vi "Bitmap File Writer.vi"   [LabVIEW 2012]
panel:
  # "观察程序框图，运行本VI。\n\n本VI没有用户界面项。"
types:
  T1 = enum16{"open", "replace", "create", "open or create", "replace or create", "replace or create with confirmation"}
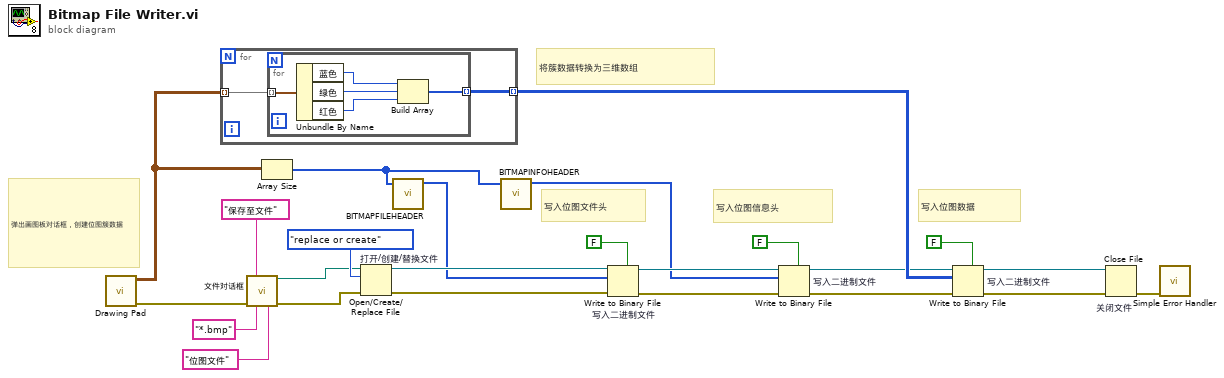
[diagram p0: block diagram]
diagram:
  # "弹出画图板对话框，创建位图簇数据"
  # "将簇数据转换为三维数组"
  # "写入位图数据"
  # "写入位图信息头"
  # "写入位图文件头"
  n1 = call "Drawing Pad.vi"() -> ("错误输出"=w4:errorcluster, "图像数据"=w14:cluster{"红色":u8, "绿色":u8, "蓝色":u8}[][])  [unwired: 10 in]
  n2 = for {
    tunnel: w14 -> [w26] mode=indexing
    tunnel: [w25] -> w12 mode=indexing
    n3 = for {
      tunnel: w26 -> [w31] mode=indexing
      tunnel: [w27] -> w25 mode=indexing
      n4 = Unbundle By Name ("按名称解除捆绑")(w31) -> ("蓝色"=w29:u8, "绿色"=w30:u8, "红色"=w28:u8)
      n5 = Build Array ("创建数组")(w29, w30, w28) -> (w27:u8[])
    }
  }
  n6 = call "文件对话框"("prompt"="保存至文件" ("提示"), "error in"=w4, "pattern (all files)"="*.bmp" ("类型（所有文件）"), "pattern label"="位图文件" ("类型标签")) -> ("selected path"=w6:path, "error out"=w5:errorcluster)  [unwired: 8 in, 2 out]
  n7 = Array Size ("数组大小")(array=w14) -> (size(s)=w17:i32[])
  n8 = Open/Create/Replace File "打开/创建/替换文件"(file path (use dialog)=w6, error in=w5, operation (0:open)=T1."replace or create" ("操作(0:open)")) -> (refnum out=w21:refnum<file>, error out=w20:errorcluster)  [unwired: 3 in, 1 out]
  n9 = call "BITMAPFILEHEADER.vi"("图像维数"=w17) -> ("位图文件头"=w16:u8[])  [unwired: 10 in]
  n10 = call "BITMAPINFOHEADER.vi"("图像维数"=w17) -> ("位图文件头"=w15:u8[])  [unwired: 10 in]
  n11 = Write to Binary File "写入二进制文件"(file (use dialog)=w21, data=w16, error in=w20, 5:FALSE ("预置数组或字符串大小？(T)")) -> (refnum out=w19:refnum<file>, error out=w18:errorcluster)  [unwired: 2 in, 1 out]
  n12 = Write to Binary File "写入二进制文件"(file (use dialog)=w19, data=w15, error in=w18, 5:FALSE ("预置数组或字符串大小？(T)")) -> (refnum out=w11:refnum<file>, error out=w10:errorcluster)  [unwired: 2 in, 1 out]
  n13 = Write to Binary File "写入二进制文件"(file (use dialog)=w11, data=w12, error in=w10, 5:FALSE ("预置数组或字符串大小？(T)")) -> (refnum out=w8:refnum<file>, error out=w9:errorcluster)  [unwired: 2 in, 1 out]
  n14 = Close File "关闭文件"(refnum=w8, error in=w9) -> (error out=w7:errorcluster)  [unwired: 1 out]
  n15 = call <vilib>:"Simple Error Handler.vi"("error in (no error)"=w7) -> ()  [unwired: 4 in, 5 out]
